vi "peak -- fit function -- arctan.vi"(3 "output control":T1, 4 "data":T2, 5 "X":dbl[](array[numeric]), 6 "a":dbl[](array[numeric])) -> (0 "error out":errorcluster, 1 "f'(X,a)":dbl[][](array[numeric]), 2 "f(X,a)":dbl[](array[numeric]))   [LabVIEW 2015]
doc: "This template is the starting point for creating a model function to be passed to the Nonlinear Curve Fit.vi."
uses:
  <vilib>/gmath/NumericalOptimization/objective function data.ctl
  <vilib>/gmath/NumericalOptimization/LM_output select.ctl
  <vilib>/gmath/NI_Gmath.lvlib
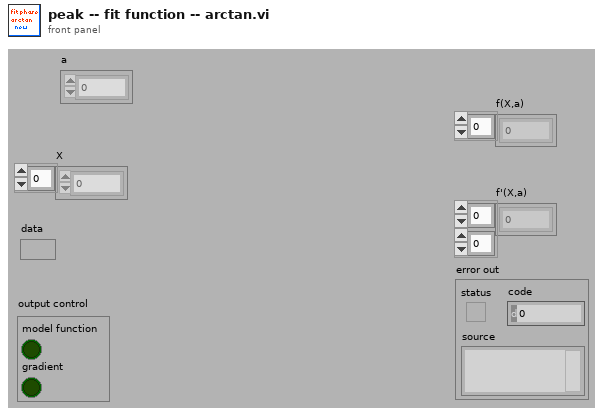
[diagram p1: front panel]
types:
  T1 = typedef "NI_Gmath.lvlib/LM_output select.ctl" = cluster{"model function":bool, "gradient":bool}
  T2 = typedef "NI_Gmath.lvlib/objective function data.ctl" = variant
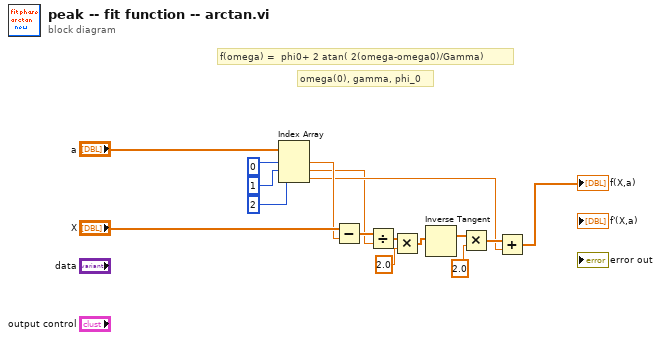
[diagram p0: block diagram]
diagram:
  # "omega(0), gamma, phi_0"
  # "f(omega) =  phi0+ 2 atan( 2(omega-omega0)/Gamma)"
  n1 = Index Array(array="a", index #1=0 ("index"), index #2=1 ("index"), index #3=2 ("index")) -> (element #1=w9:dbl, element #2=w4:dbl, element #3=w5:dbl)
  n2 = Subtract(x="X", y=w9) -> (x-y=w8:dbl[])
  n3 = Divide(x=w8, y=w4) -> (x/y=w1:dbl[])
  n4 = Multiply(x=w1, y=2.0) -> (x*y=w2:dbl[])
  n5 = Inverse Tangent(1:w2) -> (0:w7:dbl[])
  n6 = Multiply(x=w7, y=2.0) -> (x*y=w6:dbl[])
  n7 = Add(x=w6, y=w5) -> (x+y=→"f(X,a)":dbl[])
